vi "Calculate Pulse Frequency and Amplitude.vi"(11 "Waveform Array":waveform(dbl)[](array[waveform])) -> (0 "error out":errorcluster, 1 "Frequencies":dbl[](array[numeric]), 3 "Pulse Amplitudes":dbl[](array[numeric]))   [LabVIEW 2010]
uses:
  <vilib>/measure/mascope.llb/Amplitude and Levels 1 chan.vi
  <vilib>/measure/mascope.llb/Pulse Measurements 1 chan.vi
  <vilib>/measure/NI_MAPro.lvlib
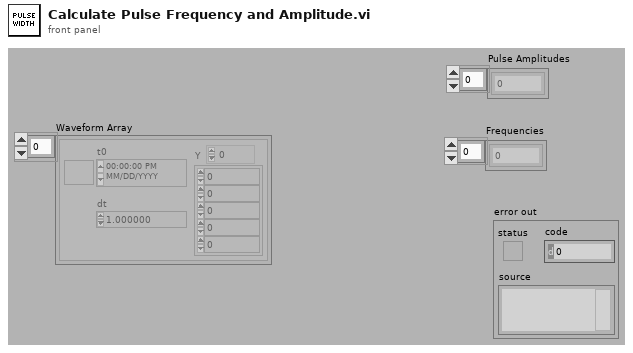
[diagram p1: front panel]
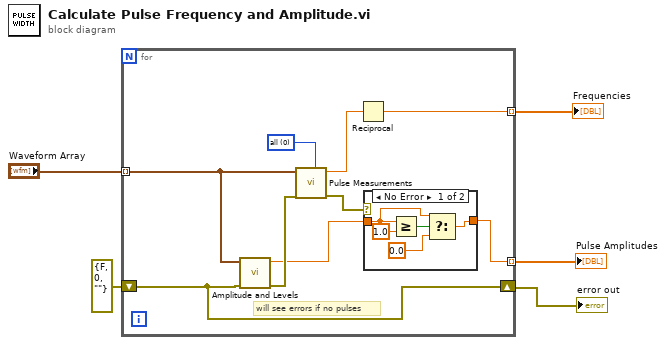
[diagram p0: block diagram]
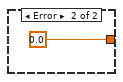
[diagram p2: hidden frame]
diagram:
  n1 = for {
    tunnel: "Waveform Array" -> [w10] mode=indexing
    tunnel: [w6] -> w1 mode=indexing
    tunnel: [w13] -> w2 mode=indexing
    shift-right: [w9] -> w4
    shift-left: errorcluster {"status"=FALSE, "code"=0, "source"=""} ("error out") -> [w9]
    w14 = u16 0 items=["all", "no period and duty cycle"] ("export mode")
    # "will see errors if no pulses"
    n2 = call-poly <vilib>:"Amplitude and Levels.vi"("error in (no error)"=w9, "signal in"=w10) -> ("error out"=w11:errorcluster, "amplitude"=w7:dbl)  [unwired: 6 in, 2 out]
    n3 = call-poly <vilib>:"Pulse Measurements.vi"("export mode"=w14, "error in (no error)"=w11, "signal in"=w10) -> ("error out"=w8:errorcluster, "period"=w12:dbl)  [unwired: 4 in, 3 out]
    n4 = Reciprocal(x=w12) -> (1/x=w13:dbl)
    n5 = case shown="No Error" w8 {
      tunnel: w7 -> [w17 _]
      tunnel: [w15 0.0 ("amplitude")] -> w6
      frame No Error {
        n6 = Greater Or Equal?(x=w17, y=1.0) -> (x >= y?=w18:bool)
        n7 = Select(t=w17, s=w18, f=0.0) -> (s? t:f=w15:dbl)
      }
      frame Error {
      }
    }
  }
  "error out" <- w4
  "Pulse Amplitudes" <- w1
  "Frequencies" <- w2
